vi "spoof_pump_control.vi"(0 "VISA resource name":refnum<visa-resource-name>="ASRL1::INSTR", 1 "Direction":u16(ring) items=["Infuse", "Withdraw", "No Action"], 2 "Syringe Inside Diameter (19.58 mm)\nIf diameter is upper than 14.00 mm : Volume units are mL\nIf diameter is lower than 14.00 mm : Volume units are µL":dbl=19.58 min=0.1 max=50.0 step=0.01 format="%#_4g", 3 "Dispense Volume (mL)":dbl=1.5 format="%_6f", 4 "Units":i32(ring)=2 items=["microliters per minute (µL/min)", "microliters per hour (µL/hr)", "milliliters per minute (mL/min)", "milliliters per hour (mL/hr)"], 5 "Flow rate":dbl=5.0 format="%.3f") -> (6 "Pump : New Era Pump Systems Inc.\nFirmware Version :":string, 7 "Volume Dispensed":string, 8 "Pump Status":T1)   [LabVIEW 2019]
panel:
  in  "Pump Address (0)":i32 format="%0#.0f"
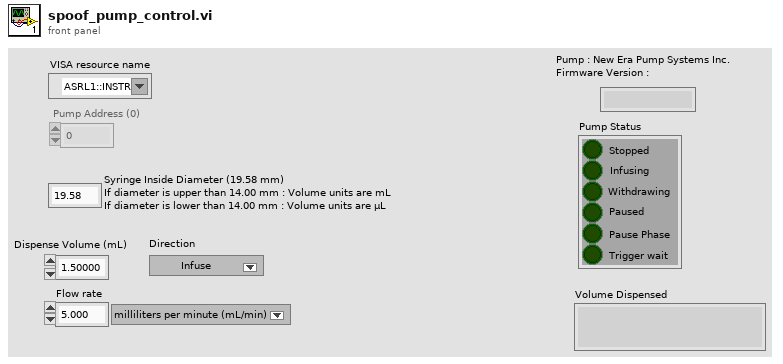
[diagram p1: front panel]
types:
  T1 = cluster{"Stopped":bool, "Infusing":bool, "Withdrawing":bool, "Paused":bool, "Pause Phase":bool, "Trigger wait":bool}
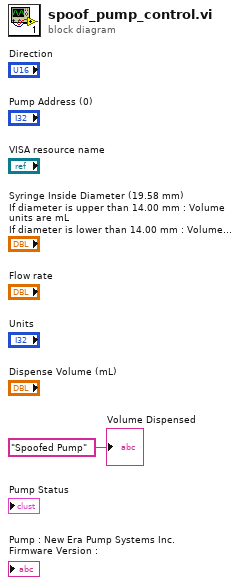
[diagram p0: block diagram]
diagram:
  "Volume Dispensed" <- "Spoofed Pump" ("Volume Dispensed")
